vi "Get topic.vi"(11 "Subscribe JSON in":refnum<class "Subscribe JSON.lvclass">) -> (2 "Topic":string, 3 "Subscribe JSON out":refnum<class "Subscribe JSON.lvclass">)   [LabVIEW 2020, in "wamplv.lvlib" / "Subscribe JSON.lvclass"]
uses:
  Subscribe JSON.lvclass
  Subscribe JSON.lvclass/Subscribe JSON.ctl
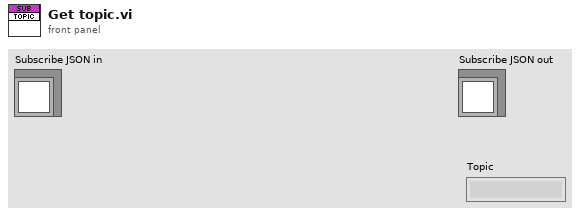
[diagram p1: front panel]
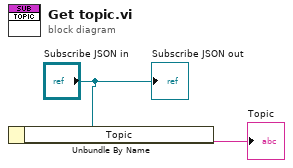
[diagram p0: block diagram]
diagram:
  n1 = Unbundle By Name("Subscribe JSON in") -> ("Topic"=→"Topic":string)
  "Subscribe JSON out" <- "Subscribe JSON in"
